vi "Least Square.vi"   [LabVIEW 2018]
doc: "VI criada para realizar o método de mínimos múltiplos quadrados para comparação do modelo real e simulado e validação do sistema"
uses:
  <vilib>/Analysis/NI_AALPro.lvlib
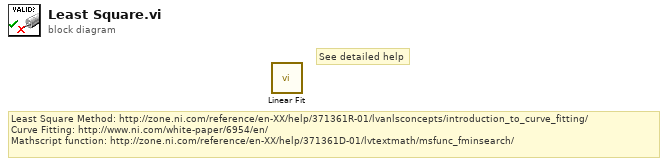
[diagram p0: block diagram]
diagram:
  # "See detailed help"
  # "Least Square Method: http://zone.ni.com/reference/en-XX/help/371361R-01/lvanlsconcepts/introduction_to_curve_fitting/\nCurve Fitting: http://www.ni.com/white-paper/6954/en/\nMathscript function: http://zone.ni.com/reference/en-XX/help/371361D-01/lvtextmath/msfunc_fminsearch/"
  n1 = call <vilib>:"Linear Fit.vi"() -> ()  [unwired: 11 in, 5 out]
